vi "ATF Storage-NS Reader.vi"(8 "error in (no error)":errorcluster) -> (0 "error IO":errorcluster, 2 "Message Data":variant, 3 "Message":string)   [LabVIEW 2022 SP3]
uses:
  ATF Storage-RT_Global_R.vi
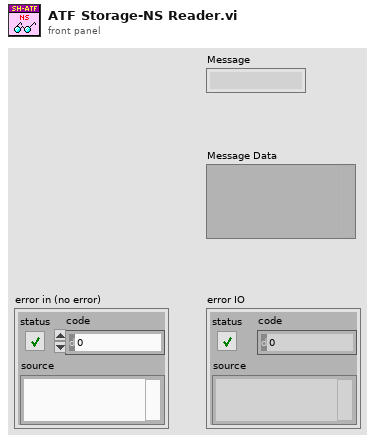
[diagram p1: front panel]
types:
  T1 = cluster{"Message":string, "Message Data":variant}
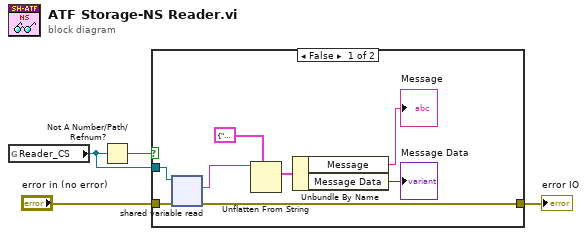
[diagram p0: block diagram]
diagram:
  n1 = global read "ATF Storage-RT_Global_R.vi" "Reader_CS"() -> (w3:refnum<k21>)
  n2 = Not A Number/Path/Refnum?(number/path/refnum=w3) -> (NaN/Path/Refnum?=w2:bool)
  n3 = case shown="False" w2 {
    tunnel: "error in (no error)" -> [w12 w13]
    tunnel: w3 -> [w11 _]
    tunnel: [w10 w13] -> w1
    frame False {
      n4 = shared-variable-read(w11, w12) -> (w10:errorcluster, w7:string)  [unwired: 1 in, 2 out]
      n5 = Unflatten From String(type=T1 {"Message"="", "Message Data"=variant} ("input cluster"), binary string=w7) -> (value=w5:T1)  [unwired: 3 in, 2 out]
      n6 = Unbundle By Name(w5) -> ("Message"=→"Message":string, "Message Data"=→"Message Data":variant)
    }
    frame True {
    }
  }
  "error IO" <- w1
